vi "LecturaCal.vi"(9 "T1":refnum<vi>) -> (0 "error out":errorcluster, 1 "Factor Potència":dbl, 3 "Nom Sensor Temperatura":string)   [LabVIEW 2017]
uses:
  <vilib>/registry/registry.llb/Registry RtKey.ctl
  <vilib>/registry/registry.llb/Read Registry Value Simple STR.vi
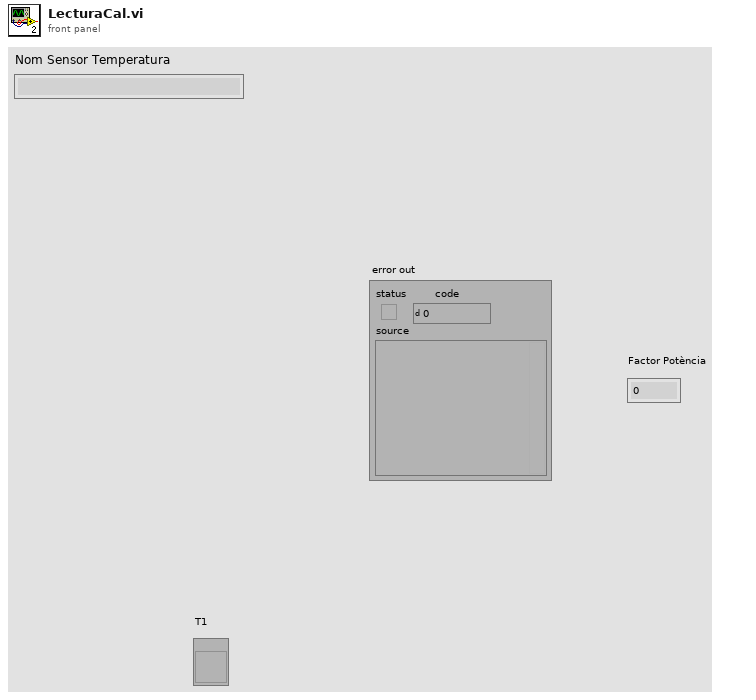
[diagram p1: front panel]
types:
  T1 = typedef "Registry RtKey.ctl" = enum32{"HKEY_CLASSES_ROOT", "HKEY_CURRENT_USER", "HKEY_LOCAL_MACHINE", "HKEY_USERS", "HKEY_PERFORMANCE_DATA", "HKEY_CURRENT_CONFIG", "HKEY_DYN_DATA"}
  T2 = typedef "Registry refnum.ctl" = refnum<k1>
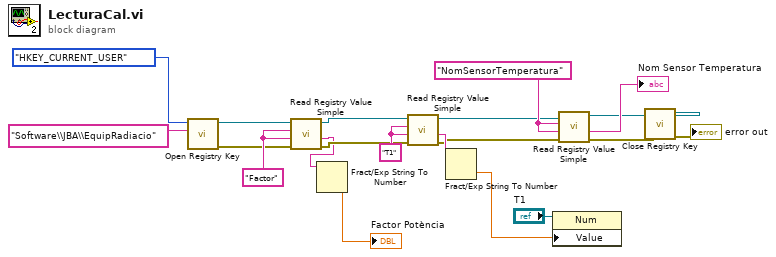
[diagram p0: block diagram]
diagram:
  w7 = "Factor" ("value")
  w13 = "NomSensorTemperatura" ("value")
  w19 = "T1" ("value")
  n1 = call <vilib>:"Open Registry Key.vi"("subkey"="Software\\JBA\\EquipRadiacio", "root key (HKEY_LOCAL_MACHINE)"=Registry_RtKey."HKEY_CURRENT_USER") -> ("error out"=w4:errorcluster, "refnum out"=w6:T2)  [unwired: 8 in]
  n2 = call-poly <vilib>:"Read Registry Value Simple.vi"("error in (no error)"=w4, "default data"=w7, "value"=w7, "refnum"=w6) -> ("error out"=w3:errorcluster, "String/Binary data"=w2:string, "refnum out"=w5:T2)  [unwired: 2 in, 1 out]
  n3 = Fract/Exp String To Number(string=w2) -> (number=→"Factor Potència":dbl)  [unwired: 3 in, 1 out]
  n4 = call-poly <vilib>:"Read Registry Value Simple.vi"("error in (no error)"=w3, "default data"=w19, "value"=w19, "refnum"=w5) -> ("error out"=w8:errorcluster, "String/Binary data"=w18:string, "refnum out"=w9:T2)  [unwired: 2 in, 1 out]
  n5 = Fract/Exp String To Number(string=w18) -> (number=w20:dbl)  [unwired: 3 in, 1 out]
  n6 = property on="Property Node" class="Num"(reference="T1", "Value"=w20) -> ()  [unwired: 1 in, 2 out]
  n7 = call-poly <vilib>:"Read Registry Value Simple.vi"("error in (no error)"=w8, "default data"=w13, "value"=w13, "refnum"=w9) -> ("error out"=w10:errorcluster, "String/Binary data"=→"Nom Sensor Temperatura":string, "refnum out"=w11:T2)  [unwired: 2 in, 1 out]
  n8 = call <vilib>:"Close Registry Key.vi"("error in (no error)"=w10, "refnum"=w11) -> ("error out"=→"error out":errorcluster)  [unwired: 5 in]
